vi "Read.vi"(7 "SPI Channel (0)":u8, 8 "Error In":errorcluster, 10 "CS Channel":u8=10, 11 "LINX Resource":T1) -> (0 "Erro Out":errorcluster, 2 "Light Level (%)":dbl, 3 "LINX Resource":T1)   [LabVIEW 2014, in "LMH-LINX.lvlib" / "PmodALS.lvlib"]
doc: "Read the arbitrary light intensity from the PmodALS (0-100)."
uses:
  <vilib>/MakerHub/LINX/Public/Sensors/Pmods/ALS/PmodALS.lvlib
  <vilib>/MakerHub/LINX/Private/Type Defs/LINX Ref.ctl
  <vilib>/MakerHub/LINX/Private/Type Defs/Platform.ctl
  <vilib>/MakerHub/LINX/Private/Type Defs/Interface.ctl
  <vilib>/MakerHub/LINX/Private/Device/Type Defs/LINX Device Config.ctl
  <vilib>/MakerHub/LINX/Private/Device/Type Defs/TCP Config.ctl
  <vilib>/MakerHub/LINX/Private/Device/Type Defs/Channels.ctl
  <vilib>/MakerHub/LINX/Public/Peripherals/SPI/SPI CS Config.ctl
  <vilib>/MakerHub/LINX/Private/Type Defs/Peripherals/SPI/SPI CS Logic Level.ctl
  <vilib>/MakerHub/LINX/Public/Peripherals/SPI/SPI Write Read 1 Frame.vi
  <vilib>/MakerHub/LINX/Public/Peripherals/SPI/SPI Write Read N Frames.vi
  <vilib>/MakerHub/LINX/Public/Utilities/Check Channel.vi
  <vilib>/MakerHub/LINX/Private/Utilties/Generate Error.vi
  <vilib>/MakerHub/LINX/LMH-LINX.lvlib
  <vilib>/MakerHub/LINX/Private/Device/Device.lvlib
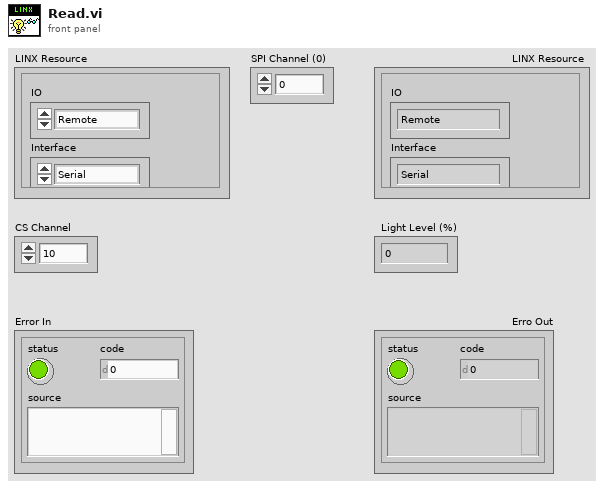
[diagram p1: front panel]
types:
  T1 = typedef "LMH-LINX.lvlib/LINX Ref.ctl" = cluster{"IO":T2, "Interface":T3, "LINX Device Config":T4}
  T2 = typedef "LMH-LINX.lvlib/Platform.ctl" = enum16{"Remote", "Local"}
  T3 = typedef "LMH-LINX.lvlib/Interface.ctl" = enum16{"Serial", "TCP"}
  T4 = typedef "LMH-LINX.lvlib/Device.lvlib/LINX Device Config.ctl" = cluster{"Interface":T3, "COM Port":refnum<visa-resource-name>, "TCP Configuration":T5, "Device Family":u8, "Device ID":u8, "Device Name":string, "TCP Ref":refnum<k5>, "Channels":T6}
  T5 = typedef "LMH-LINX.lvlib/Device.lvlib/TCP Config.ctl" = cluster{"IP Address":string, "Port":u16}
  T6 = typedef "LMH-LINX.lvlib/Channels.ctl" = cluster{"DI":u8[], "DO":u8[], "AI":u8[], "AO":u8[], "PWM":u8[], "QE":u8[], "UART":u8[], "I2C 2":u8[], "SPI":u8[], "CAN":u8[], "Servo":u8[], "AI Ref (V)":dbl, "AI Resolution (Bits)":u8, "AO Ref (V)":dbl, "AO Resolution (Bits)":u8}
  T7 = typedef "LMH-LINX.lvlib/SPI CS Config.ctl" = cluster{"CS Channel":u8, "CS Logic Level":T8}
  T8 = typedef "LMH-LINX.lvlib/SPI CS Logic Level.ctl" = enum8{"Active Low", "Active High"}
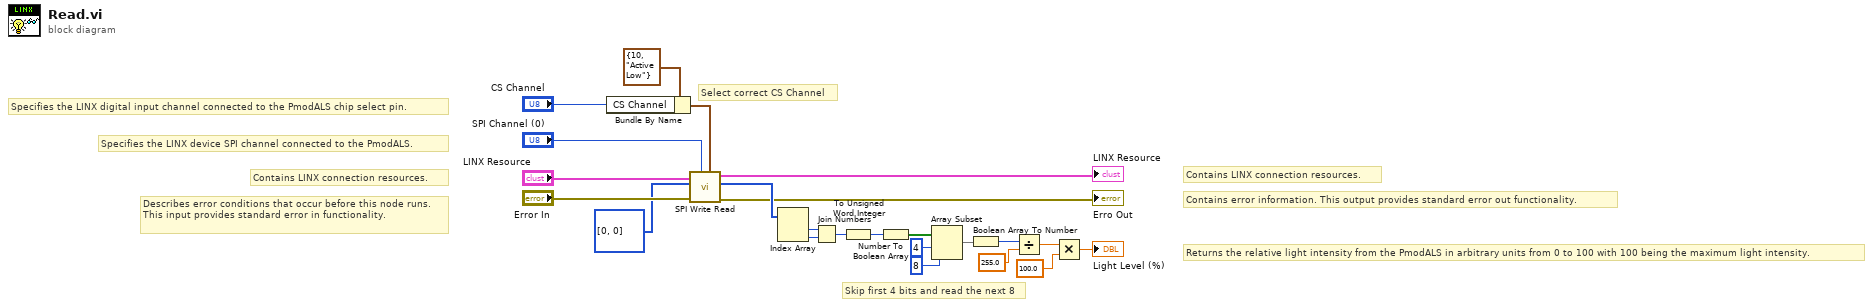
[diagram p0: block diagram]
diagram:
  # "Specifies the LINX device SPI channel connected to the PmodALS."
  # "Specifies the LINX digital input channel connected to the PmodALS chip select pin."
  # "Returns the relative light intensity from the PmodALS in arbitrary units from 0 to 100 with 100 being the maximum light intensity."
  # "Contains LINX connection resources."
  # "Contains error information. This output provides standard error out functionality."
  # "Contains LINX connection resources."
  # "Describes error conditions that occur before this node runs. This input provides standard error in functionality."
  # "Skip first 4 bits and read the next 8"
  # "Select correct CS Channel"
  n1 = Bundle By Name(cluster=T7 {"CS Channel"=10, "CS Logic Level"=enum."Active Low"} ("CS Configuration"), "CS Channel"="CS Channel") -> (w2:T7)
  n2 = call-poly <vilib>:"SPI Write Read.vi"("CS Configuration"=w2, "SPI Channel (0)"="SPI Channel (0)", "Error In"="Error In", "Data"=u8[] [0, 0], "LINX Resource"="LINX Resource") -> ("Error Out"=→"Erro Out":errorcluster, "Read Data"=w22:u8[], "LINX Resource"=→"LINX Resource":T1)  [unwired: 4 in]
  n3 = Index Array(array=w22) -> (element #1=w12:u8, element #2=w13:u8)  [unwired: 2 in]
  n4 = Join Numbers(hi=w12, lo=w13) -> ((hi.lo)=w11:u16)
  n5 = To Unsigned Word Integer(number=w11) -> (unsigned 16bit integer=w14:u16)
  n6 = Number To Boolean Array(number=w14) -> (Boolean array=w15:bool[])
  n7 = Array Subset(array=w15, index=4, length=8) -> (w18:bool[])
  n8 = Boolean Array To Number(Boolean array=w18) -> (number=w23:u32)
  n9 = Divide(x=w23, y=255.0) -> (x/y=w20:dbl)
  n10 = Multiply(x=w20, y=100.0) -> (x*y=→"Light Level (%)":dbl)
